vi "moveFilterWheel.vi"(8 "error in (no error)":errorcluster, 10 "Filter Wheel Position":u8, 11 "SpectrographClientCommunicator in":refnum<class "SpectrographClientCommunicator.lvclass">) -> (0 "error out":errorcluster, 3 "SpectrographClientCommunicator out":refnum<class "SpectrographClientCommunicator.lvclass">)   [LabVIEW 2016, in "SpectrographClientCommunicator.lvclass"]
uses:
  SpectrographClientCommunicator.lvclass
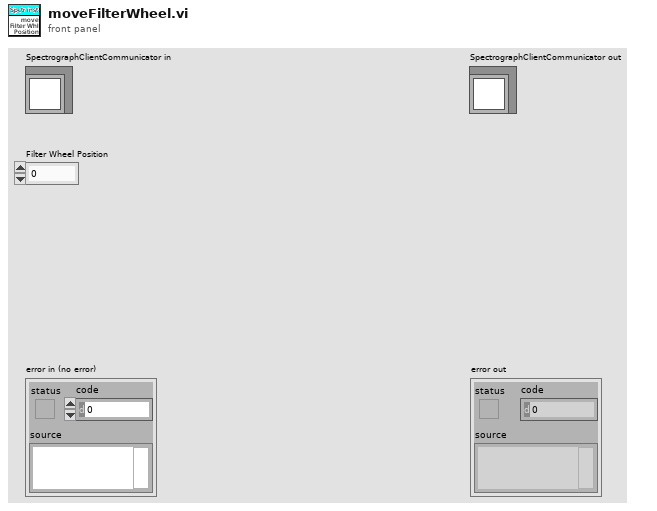
[diagram p1: front panel]
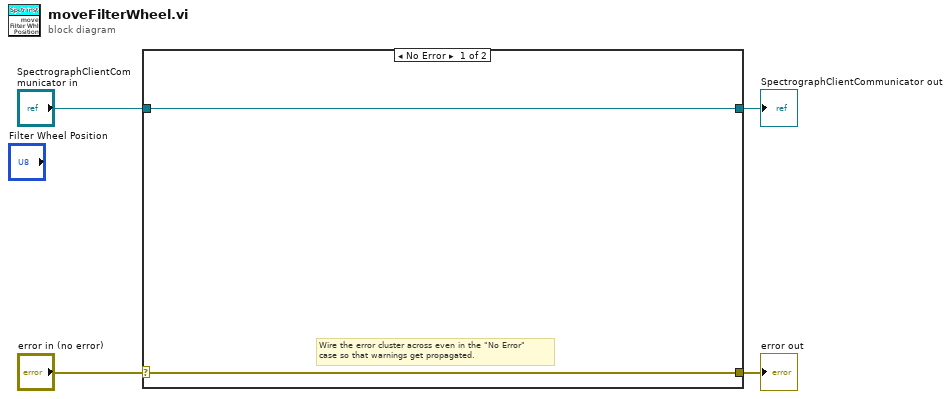
[diagram p0: block diagram]
diagram:
  n1 = case shown="No Error" "error in (no error)" {
    selector: "error in (no error)" -> [w5 w8]
    tunnel: [w5 w8] -> w3
    tunnel: [w6 w7] -> w1
    tunnel: "SpectrographClientCommunicator in" -> [w6 w7]
    frame No Error {
      # "Wire the error cluster across even in the \"No Error\"\ncase so that warnings get propagated."
    }
    frame Error {
    }
  }
  "error out" <- w3
  "SpectrographClientCommunicator out" <- w1
